vi "忽略错误-网络超时.vi"(8 "错误输入":errorcluster caption="输入簇") -> (0 "错误输出":errorcluster)   [LabVIEW 2017]
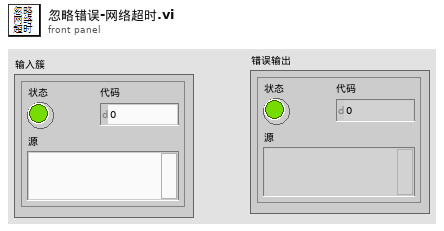
[diagram p1: front panel]
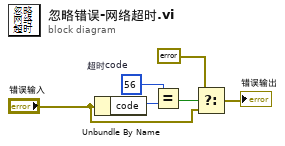
[diagram p0: block diagram]
diagram:
  w5 = 56  # 超时code
  n1 = Unbundle By Name("错误输入") -> ("code"=w6:i32)
  n2 = Equal?(x=w5, y=w6) -> (x = y?=w4:bool)
  n3 = Select(t=errorcluster {"status"=FALSE, "code"=0, "source"=""}, s=w4, f="错误输入") -> (s? t:f=→"错误输出":errorcluster)
